vi "tsapp_receive_can_message_win32.vi"(8 "错误输入（无错误）":errorcluster, 9 "AOnlyRx":u8, 10 "AAppChannel输入":i32) -> (0 "错误输出":errorcluster, 1 "tsapp_receive_can_message":bool, 4 "Receive message":T1)   [LabVIEW 2010]
uses:
  SendMsgInfo.ctl
  MessageInfo.ctl
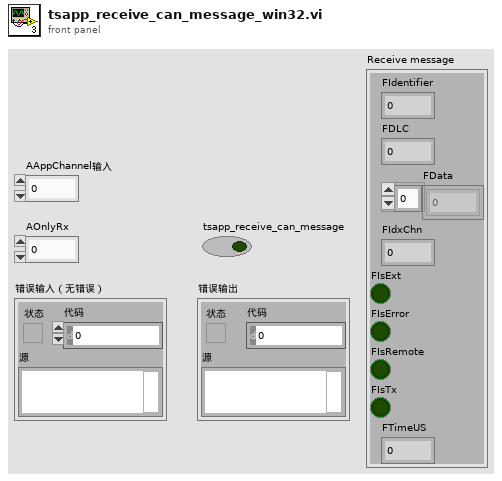
[diagram p1: front panel]
types:
  T1 = typedef "MessageInfo.ctl" = cluster{"FIdentifier":i32, "FDLC":u8, "FData":u8[], "FIdxChn":u8, "FIsExt":bool, "FIsError":bool, "FIsRemote":bool, "FIsTx":bool, "FTimeUS":u64}
  T2 = typedef "SendMsgInfo.ctl" = cluster{"FIdxChn":u8, "FProperties":u8, "FDLC":u8, "FReserved":u8, "FIdentifier":i32, "FTimeUS":u64, "Data0":u8, "Data1":u8, "Data2":u8, "Data3":u8, "Data4":u8, "Data5":u8, "Data6":u8, "Data7":u8}
  T3 = typedef "TCANProperty.ctl" = cluster{"istx":bool, "remoteframe":bool, "extframe":bool, "tbd1":bool, "tbd2":bool, "tbd3":bool, "tbd4":bool, "iserrorframe":bool}
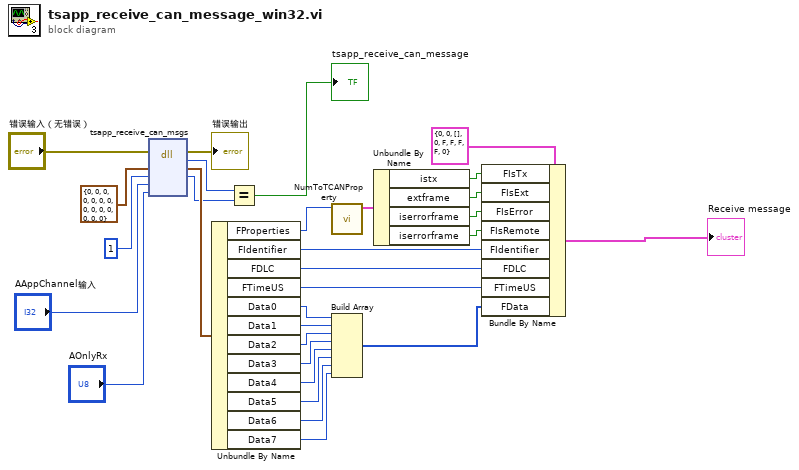
[diagram p0: block diagram]
diagram:
  n1 = dll-call lib="PTH1`abs DLabviewWorkSpace海卓项目资料\tHaiDriverBottomLevelTS_CANDriveTSMaster.dll" fn="tsapp_receive_can_msgs"(error in="错误输入（无错误）", "ACANBuffers"=T2 {"FIdxChn"=0, "FProperties"=0, "FDLC"=0, "FReserved"=0, "FIdentifier"=0, "FTimeUS"=0, "Data0"=0, "Data1"=0, "Data2"=0, "Data3"=0, "Data4"=0, "Data5"=0, "Data6"=0, "Data7"=0} ("SendMsgInfo"), "ACANBufferSize"=1, "AChn"="AAppChannel输入", "ARxTx"="AOnlyRx") -> (error out=→"错误输出":errorcluster, "tsapp_receive_can_msgs"=w3:i32, "ACANBuffers"=w22:T2, "ACANBufferSize"=w1:i32)  [unwired: 4 in, 1 out]
  n2 = Unbundle By Name(w22) -> ("FProperties"=w21:u8, "FIdentifier"=w15:i32, "FDLC"=w14:u8, "FTimeUS"=w13:u64, "Data0"=w12:u8, "Data1"=w11:u8, "Data2"=w10:u8, "Data3"=w9:u8, "Data4"=w8:u8, "Data5"=w7:u8, "Data6"=w6:u8, "Data7"=w5:u8)
  n3 = Equal?(x=w3, y=w1) -> (x = y?=→"tsapp_receive_can_message":bool)
  n4 = call "NumToTCANProperty.vi"("TCANPropertyNum"=w21) -> ("TCANProperty"=w20:T3)  [unwired: 10 in]
  n5 = Build Array(w12, w11, w10, w9, w8, w7, w6, w5) -> (w4:u8[])
  n6 = Unbundle By Name(w20) -> ("istx"=w19:bool, "extframe"=w18:bool, "iserrorframe"=w17:bool, "iserrorframe"=w16:bool)
  n7 = Bundle By Name(cluster=T1 {"FIdentifier"=0, "FDLC"=0, "FData"=[], "FIdxChn"=0, "FIsExt"=FALSE, "FIsError"=FALSE, "FIsRemote"=FALSE, "FIsTx"=FALSE, "FTimeUS"=0} ("Receive message"), "FIsTx"=w19, "FIsExt"=w18, "FIsError"=w17, "FIsRemote"=w16, "FIdentifier"=w15, "FDLC"=w14, "FTimeUS"=w13, "FData"=w4) -> (→"Receive message":T1)
